vi "Load String Array.vi"(7 "section":string, 8 "error in (no error)":errorcluster, 10 "key":string, 11 "refnum":T1) -> (0 "error out":errorcluster, 1 "String Array Out":string[](array[string]), 3 "refnum out":T1)   [LabVIEW 2009]
uses:
  <vilib>/Utility/config.llb/Config Data RefNum.ctl
  <vilib>/Utility/config.llb/Read Key (String).vi
  <vilib>/Utility/config.llb/NI_LVConfig.lvlib
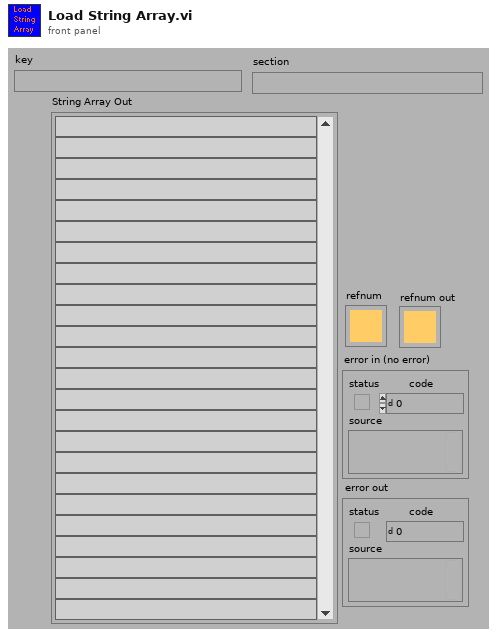
[diagram p1: front panel]
types:
  T1 = typedef "NI_LVConfig.lvlib/Config Data RefNum.ctl" = refnum<k1>
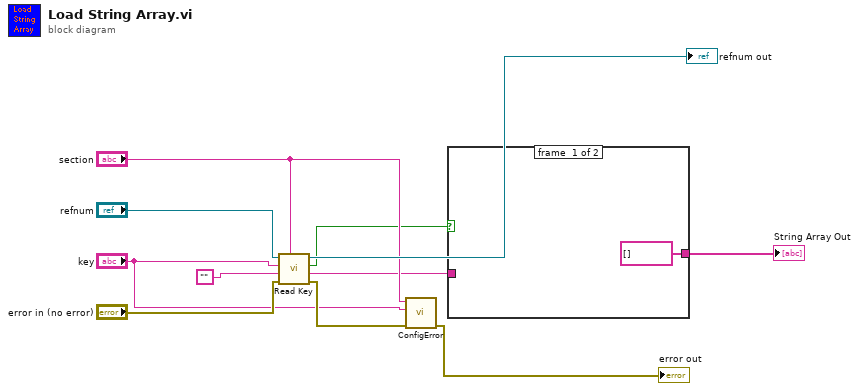
[diagram p0: block diagram]
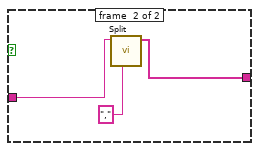
[diagram p2: hidden frame]
diagram:
  n1 = call-poly <vilib>:"Read Key.vi"("section"="section", "error in (no error)"="error in (no error)", "default value"="", "key"="key", "refnum"="refnum") -> ("error out"=w7:errorcluster, "value"=w2:string, "found?"=w3:bool, "refnum out"=→"refnum out":T1)  [unwired: 1 in, 2 out]
  n2 = call "ConfigError.vi"("error in (no error)"=w7, "Key"="key", "Section"="section") -> ("error out"=→"error out":errorcluster)  [unwired: 8 out]
  n3 = case shown="True" w3 {
    tunnel: w2 -> [_ w15]
    tunnel: [string[] [] ("Array Result") w14] -> w1
    frame #0 {
    }
    frame #1 {
      n4 = call "Split.vi"("delimiter"=",", "String"=w15) -> ("Array Result"=w14:string[])  [unwired: 9 out]
    }
  }
  "String Array Out" <- w1
